vi "MicroGear NETPIE Demo.vi"   [LabVIEW 2014]
uses:
  QwaveSys_ESP8266/QwaveSys_ESP8266.lvlib
  QwaveSys_Microgear/QwaveSys_Microgear.lvlib
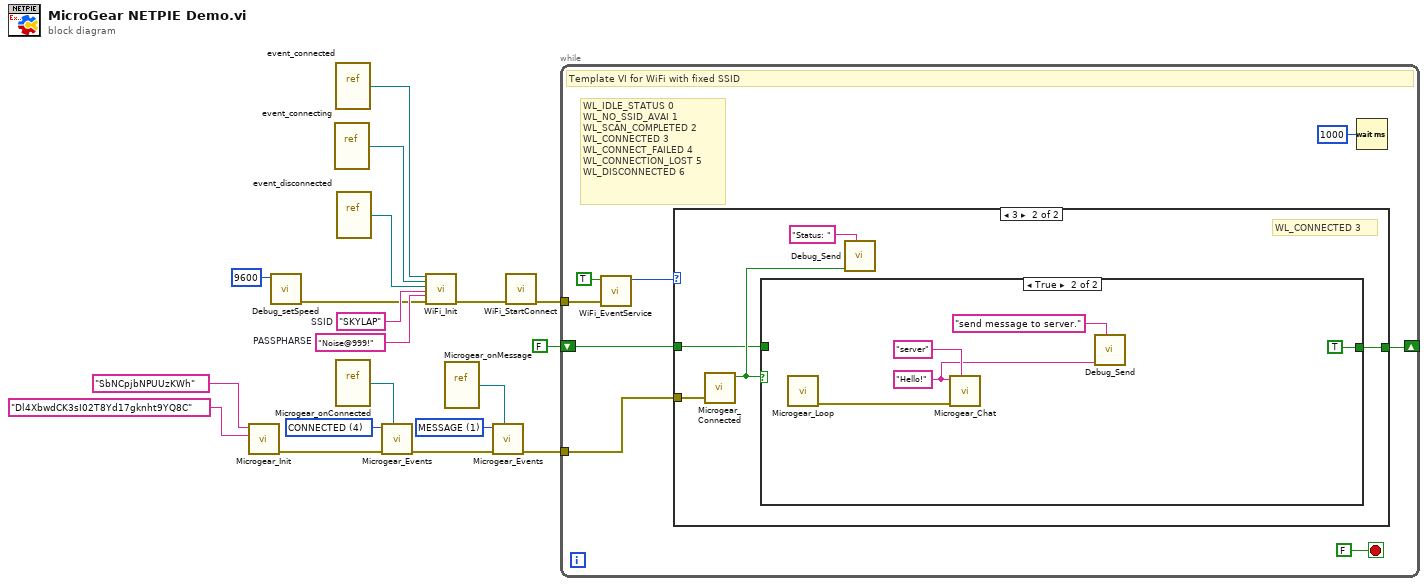
[diagram p0: block diagram]
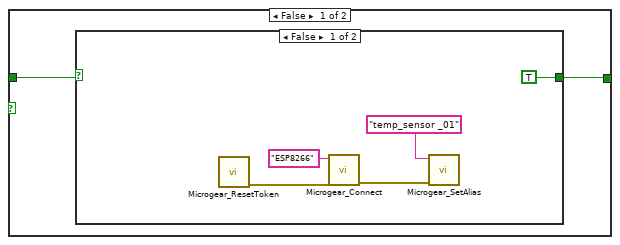
[diagram p3: hidden frame]
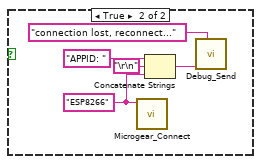
[diagram p4: hidden frame]
diagram:
  w2 = u8 1 items=["MESSAGE"=1, "PRESENT"=2, "ABSENT"=3, "CONNECTED"=4] ("events")
  w10 = u8 4 items=["MESSAGE"=1, "PRESENT"=2, "ABSENT"=3, "CONNECTED"=4] ("events")
  w18 = "Noise@999!"  # PASSPHARSE
  w17 = "SKYLAP"  # SSID
  n1 = call "Microgear_Init.vi"("SECRET"="Dl4XbwdCK3sI02T8Yd17gknht9YQ8C", "KEY"="SbNCpjbNPUUzKWh") -> ("error out"=w5:errorcluster)  [unwired: 9 in]
  n2 = call "Debug_setSpeed.vi"("Speed"=u32 9600) -> ("error out"=w16:errorcluster)  [unwired: 10 in]
  n3 = vi-ref "event_connecting.vi"() -> (w12:refnum<vi>)
  n4 = vi-ref "event_connected.vi"() -> (w13:refnum<vi>)
  n5 = vi-ref "Microgear_onConnected.vi"() -> (w9:refnum<vi>)
  n6 = vi-ref "event_disconnected.vi"() -> (w14:refnum<vi>)
  n7 = call "Microgear_Events.vi"("function"=w9, "error in (no error)"=w5, "events"=w10) -> ("error out"=w4:errorcluster)  [unwired: 8 in]
  n8 = call "WiFi_Init.vi"("connected"=w13, "connecting"=w12, "disconnected"=w14, "SSID"=w17, "PASSPHARSE"=w18, "error in (no error)"=w16) -> ("error out"=w15:errorcluster)  [unwired: 9 in]
  n9 = vi-ref "Microgear_onMessage.vi"() -> (w1:refnum<vi>)
  n10 = call "Microgear_Events.vi"("function"=w1, "error in (no error)"=w4, "events"=w2) -> ("error out"=w3:errorcluster)  [unwired: 8 in]
  n11 = call "WiFi_StartConnect.vi"("error in (no error)"=w15) -> ("error out"=w11:errorcluster)  [unwired: 10 in]
  n12 = while {
    tunnel: w11 -> [w26]
    tunnel: w3 -> [w20]
    shift-right: [w21] -> _
    shift-left: FALSE ("wait for connected (True)") -> [w22]
    stop <- FALSE stop-if-true
    # "WL_IDLE_STATUS\t0\nWL_NO_SSID_AVAI\t1\nWL_SCAN_COMPLETED\t2\nWL_CONNECTED\t3\nWL_CONNECT_FAILED\t4\nWL_CONNECTION_LOST\t5\nWL_DISCONNECTED\t6"
    # "Template VI for WiFi with fixed SSID"
    n13 = call "WiFi_EventService.vi"("error in (no error)"=w26, "wait for connected (True)"=TRUE) -> ("Status"=w23:u16)  [unwired: 8 in, 1 out]
    n14 = case shown="3" w23 {
      tunnel: w20 -> [_ w32]
      tunnel: w22 -> [_ w29]
      tunnel: [_ w28] -> w21
      frame 0, Default {
        # "DISCONNECTED or default status"
      }
      frame 3 {
        # "WL_CONNECTED\t3"
        n15 = call "Microgear_Connected.vi"("error in (no error)"=w32) -> ("connected"=w31:bool)  [unwired: 9 in, 1 out]
        n16 = case shown="True" w31 {
          tunnel: w29 -> [w34 _]
          tunnel: [w33 TRUE ("wait for connected (True)")] -> w28
          frame False {
            n17 = case shown="False" w34 {
              tunnel: [TRUE ("wait for connected (True)") _] -> w33
              frame False {
                n18 = call "Microgear_ResetToken.vi"() -> ("error out"=w36:errorcluster)  [unwired: 11 in]
                n19 = call "Microgear_Connect.vi"("error in (no error)"=w36, "APPID"="ESP8266") -> ("error out"=w35:errorcluster)  [unwired: 9 in]
                n20 = call "Microgear_SetAlias.vi"("error in (no error)"=w35, "alias"="temp_sensor _01") -> ()  [unwired: 9 in, 1 out]
              }
              frame True {
                w42 = "ESP8266" ("APPID")
                n21 = call "Microgear_Connect.vi"("APPID"=w42) -> ()  [unwired: 10 in, 1 out]
                n22 = Concatenate Strings("APPID: " ("string"), "\r\n" ("End of Line Constant"), w42) -> (w43:string)
                n23 = call "Debug_Send.vi"("Name"="connection lost, reconnect...", "DATA"=w43) -> ()  [unwired: 10 in]
              }
            }
          }
          frame True {
            w47 = "Hello!" ("message")
            n24 = call "Microgear_Loop.vi"() -> ("error out"=w46:errorcluster)  [unwired: 11 in]
            n25 = call "Microgear_Chat.vi"("name"="server", "error in (no error)"=w46, "message"=w47) -> ()  [unwired: 8 in, 1 out]
            n26 = call "Debug_Send.vi"("Name"="send message to server.", "DATA"=w47) -> ()  [unwired: 10 in]
          }
        }
        n27 = call "Debug_Send.vi"("Name"="Status: ", "DATA"=w31) -> ()  [unwired: 10 in]
      }
    }
    n28 = Wait (ms)(milliseconds to wait=u32 1000) -> ()  [unwired: 1 out]
  }
